vi "request.vi"(7 "LabVIEW Web Service Request":refnum<class "Web Request.lvclass">) -> ()   [LabVIEW 2017]
uses:
  <vilib>/wsapi/Web Request.lvclass
  <vilib>/NI/NI JSONRPC Server Framework/Classes/Server/JSONRPC Server.lvclass
  <vilib>/NI/NI JSONRPC Server Framework/Classes/error/error.lvclass
  <vilib>/NI/JSON Support for LabVIEW/JSON Value/Object/Get Value/Get Value (String).vi
  <vilib>/NI/NI JSONRPC Server Framework/Classes/Server/Send Request (Sync).vi
  <vilib>/NI/NI JSONRPC Server Framework/Classes/error/error.Write code.vi
  <vilib>/NI/NI JSONRPC Server Framework/Classes/error/error.Write message.vi
  <vilib>/NI/NI JSONRPC Server Framework/Classes/error/error.Write data.vi
  <vilib>/NI/JSON Support for LabVIEW/JSON Value/JSON Value.lvclass
  <vilib>/NI/JSON Support for LabVIEW/JSON Variant Support/JSON Variant Support.lvclass
panel:
  out "error out":errorcluster
  # "Use the Web Service Request input terminal to call the VIs on the Web Services palette. Do not remove it from the connector pane unless you don't need access to the palette."
  # "Each additional control wired to the connector pane will be available as an input in the URL. To include an indicator in terminal-mode output (the default setting), it must also be wired to the connector pane."
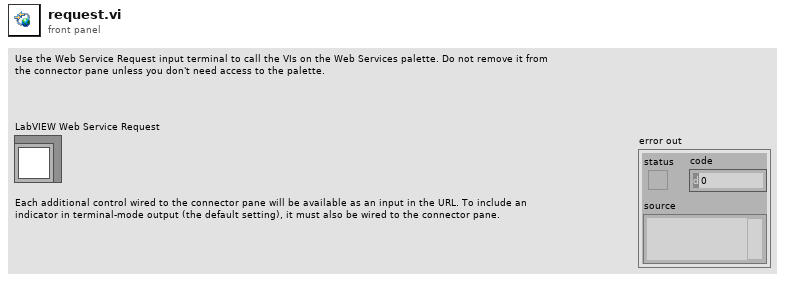
[diagram p1: front panel]
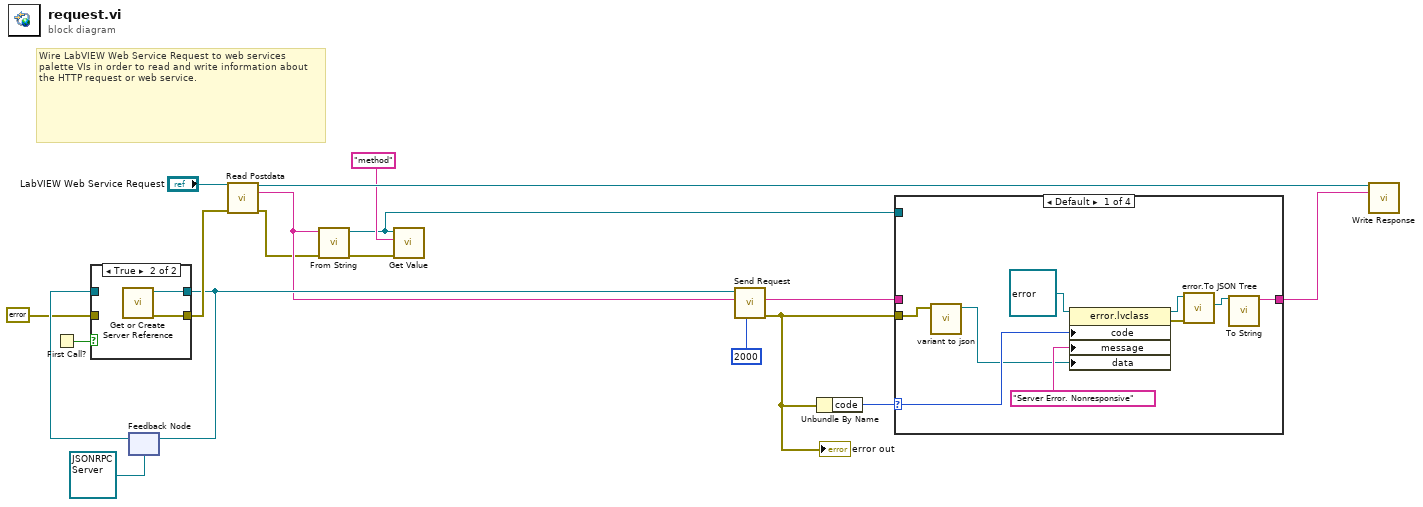
[diagram p0: block diagram]
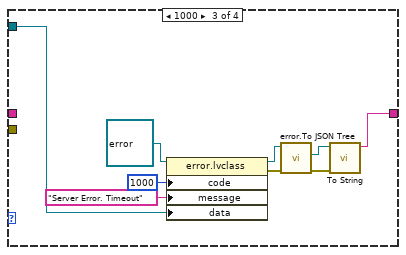
[diagram p3: hidden frame]
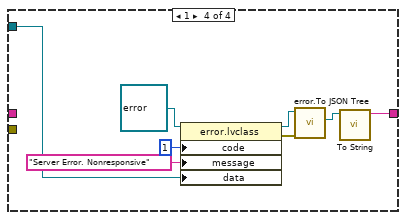
[diagram p4: hidden frame]
diagram:
  # "Wire LabVIEW Web Service Request to web services palette VIs in order to read and write information about the HTTP request or web service."
  n1 = First Call?() -> (First Call?: T/F=w16:bool)
  n2 = feedback #1(refnum<class "JSONRPC Server.lvclass"> refnum ("Server Out")) -> (w15:refnum<class "JSONRPC Server.lvclass">)
  n3 = case shown="True" w16 {
    tunnel: [w19 w22] -> w13
    tunnel: [w20 w21] -> w11
    tunnel: w15 -> [w20 _]
    tunnel: errorcluster {"status"=FALSE, "code"=0, "source"=""} ("error out") -> [w19 _]
    frame False {
    }
    frame True {
      n4 = call <vilib>:"Get or Create Server Reference.vi"() -> ("error out"=w22:errorcluster, "Server Out"=w21:refnum<class "JSONRPC Server.lvclass">)  [unwired: 10 in]
    }
  }
  n5 = feedback-in #1(w11) -> ()
  n6 = call <vilib>:"Read Postdata.vi"("LabVIEW Web Service Request"="LabVIEW Web Service Request", "error in (no error)"=w13) -> ("LabVIEW Web Service Request out"=w17:refnum<class "Web Request.lvclass">, "postdata"=w6:string, "error out"=w5:errorcluster)  [unwired: 11 in]
  n7 = call <vilib>:"From String.vi"("error in (no error)"=w5, "JSON String"=w6) -> ("error out"=w4:errorcluster, "JSON Value out"=w2:refnum<class "JSON Value.lvclass">)  [unwired: 8 in]
  n8 = call-poly <vilib>:"Get Value.vi"("error in (no error)"=w4, "key"="method", "JSON Value in"=w2) -> ()  [unwired: 7 in, 2 out]
  n9 = call-poly <vilib>:"Send Request.vi"("Timeout (-1)"=2000, "JSON Request String"=w6, "JSONRPC Server in"=w11) -> ("error out"=w1:errorcluster, "JSON Response String"=w8:string)  [unwired: 6 in, 1 out]
  "error out" <- w1
  n10 = Unbundle By Name(w1) -> ("code"=w9:i32)
  n11 = case shown="Default" w9 {
    selector: w9 -> [w25 _ _ _]
    tunnel: w8 -> [_ w32 _ _]
    tunnel: [w26 w32 w33 w43] -> w7
    tunnel: w2 -> [_ _ w36 w42]
    tunnel: w1 -> [w24 _ _ _]
    frame Default {
      n12 = call <vilib>:"variant to json.vi"("Variant"=w24) -> ("JSON Value"=w23:refnum<class "JSON Value.lvclass">)  [unwired: 9 in, 1 out]
      n13 = property class="error.lvclass"(reference=refnum<class "error.lvclass"> refnum ("error.lvclass"), "code"=w25, "message"="Server Error. Nonresponsive", "data"=w23) -> (reference out=w28:refnum<class "error.lvclass">, error out=w31:errorcluster)  [unwired: 1 in]
      n14 = call <vilib>:"error.To JSON Tree.vi"("error in (no error)"=w31, "error in"=w28) -> ("JSON Value out"=w27:refnum<class "JSON Value.lvclass">)  [unwired: 7 in, 2 out]
      n15 = call <vilib>:"To String.vi"("JSON Value in"=w27) -> ("String"=w26:string)  [unwired: 9 in, 1 out]
    }
    frame 0 {
    }
    frame 1000 {
      n16 = property class="error.lvclass"(reference=refnum<class "error.lvclass"> refnum ("error.lvclass"), "code"=1000, "message"="Server Error. Timeout", "data"=w36) -> (reference out=w37:refnum<class "error.lvclass">, error out=w41:errorcluster)  [unwired: 1 in]
      n17 = call <vilib>:"error.To JSON Tree.vi"("error in (no error)"=w41, "error in"=w37) -> ("error out"=w35:errorcluster, "JSON Value out"=w34:refnum<class "JSON Value.lvclass">)  [unwired: 7 in, 1 out]
      n18 = call <vilib>:"To String.vi"("error in (no error)"=w35, "JSON Value in"=w34) -> ("String"=w33:string)  [unwired: 8 in, 1 out]
    }
    frame 1 {
      n19 = property class="error.lvclass"(reference=refnum<class "error.lvclass"> refnum ("error.lvclass"), "code"=1, "message"="Server Error. Nonresponsive", "data"=w42) -> (reference out=w45:refnum<class "error.lvclass">, error out=w49:errorcluster)  [unwired: 1 in]
      n20 = call <vilib>:"error.To JSON Tree.vi"("error in (no error)"=w49, "error in"=w45) -> ("JSON Value out"=w44:refnum<class "JSON Value.lvclass">)  [unwired: 7 in, 2 out]
      n21 = call <vilib>:"To String.vi"("JSON Value in"=w44) -> ("String"=w43:string)  [unwired: 9 in, 1 out]
    }
  }
  n22 = call <vilib>:"Write Response.vi"("LabVIEW Web Service Request"=w17, "response string"=w7) -> ()  [unwired: 12 in, 2 out]
